vi "Uninit.vi"(11 "MQTT-Server in":refnum<class "MQTT-Server.lvclass">) -> (3 "MQTT-Server out":refnum<class "MQTT-Server.lvclass">)   [LabVIEW 2023, in "MQTT-Server.lvlib" / "MQTT-Server.lvclass"]
doc: "This method is the inverse of the Pre Launch Init.vi. This method is called unconditionally at the end of an actor's lifetime, even if there was an error in Pre Launch Init.vi. Note that the self Enqueuer for the actor is already invalid by the time this VI executes: within this method, the actor may send messages to its caller but not to itself. This method executes before Last Ack is sent.\n\nThis method neither receives nor produces an error cluster. It is designed to provide an unconditional release of acquired resources. Any error raised during release is considered to be irrelevant to the actor's lifetime. If the actor truly needs to report some error status, it may send a message to caller or include information within itself that callers can examine when handling Last Ack."
uses:
  MQTT-Server.lvclass
  MQTT-Server.lvclass/MQTT-Server.ctl
  <vilib>/ActorFramework/Actor/Actor.lvclass
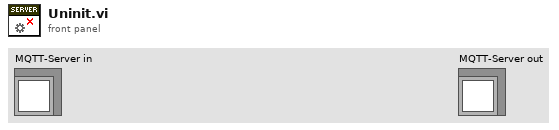
[diagram p1: front panel]
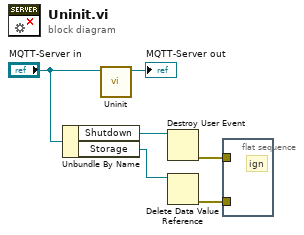
[diagram p0: block diagram]
diagram:
  n1 = Unbundle By Name("MQTT-Server in") -> ("Shutdown"=w4:refnum<user-event>, "Storage"=w2:refnum<data-value>)
  n2 = call-parent "Uninit.vi"("Actor in"="MQTT-Server in") -> ("Actor out"=→"MQTT-Server out":refnum<class "MQTT-Server.lvclass">)  [unwired: 10 in]
  n3 = Destroy User Event(user event=w4) -> (error out=w3:errorcluster)  [unwired: 1 in]
  n4 = Delete Data Value Reference(data value reference=w2) -> (error out=w1:errorcluster)  [unwired: 1 in, 1 out]
  n5 = flat-sequence {
    tunnel: w3 -> [_]
    tunnel: w1 -> [_]
    frame #0 {
      # "ign"
    }
  }
